vi "get ema report data from imei list file.vi"(8 "error in (no error)":errorcluster) -> (0 "error out":errorcluster, 2 "Rec count":i32, 3 "Array":string[][](array[string]))   [LabVIEW 2013]
uses:
  <vilib>/Utility/file.llb/Read From Spreadsheet File (string).vi
  <vilib>/Utility/file.llb/Write To Spreadsheet File (string).vi
panel:
  in  "Array 2":string[][](array[string])=[["partNumber", "revNumber", "Imei", "Serial", "deviceId", "mfgSerial", "testTimestamp", "simId1", "simId2", "VZWFW", "ATTFW", "moduleBuildVer", "model"]]
  in  "SQL Query":string="SELECT part_number AS partNumber,[PN Rev] AS revNumber,imei AS Imei,deviceserialnumber AS Serial,deviceid0 AS deviceId,btw_sn AS mfgSerial,date_time AS testTimestamp,simid1 AS simId1,simid2 AS simId2,firmware_rev AS VZWFW,deviceid1 AS ATTFW,appfwver AS moduleBuildver,devicename AS model FROM test_data WHERE imei = '"
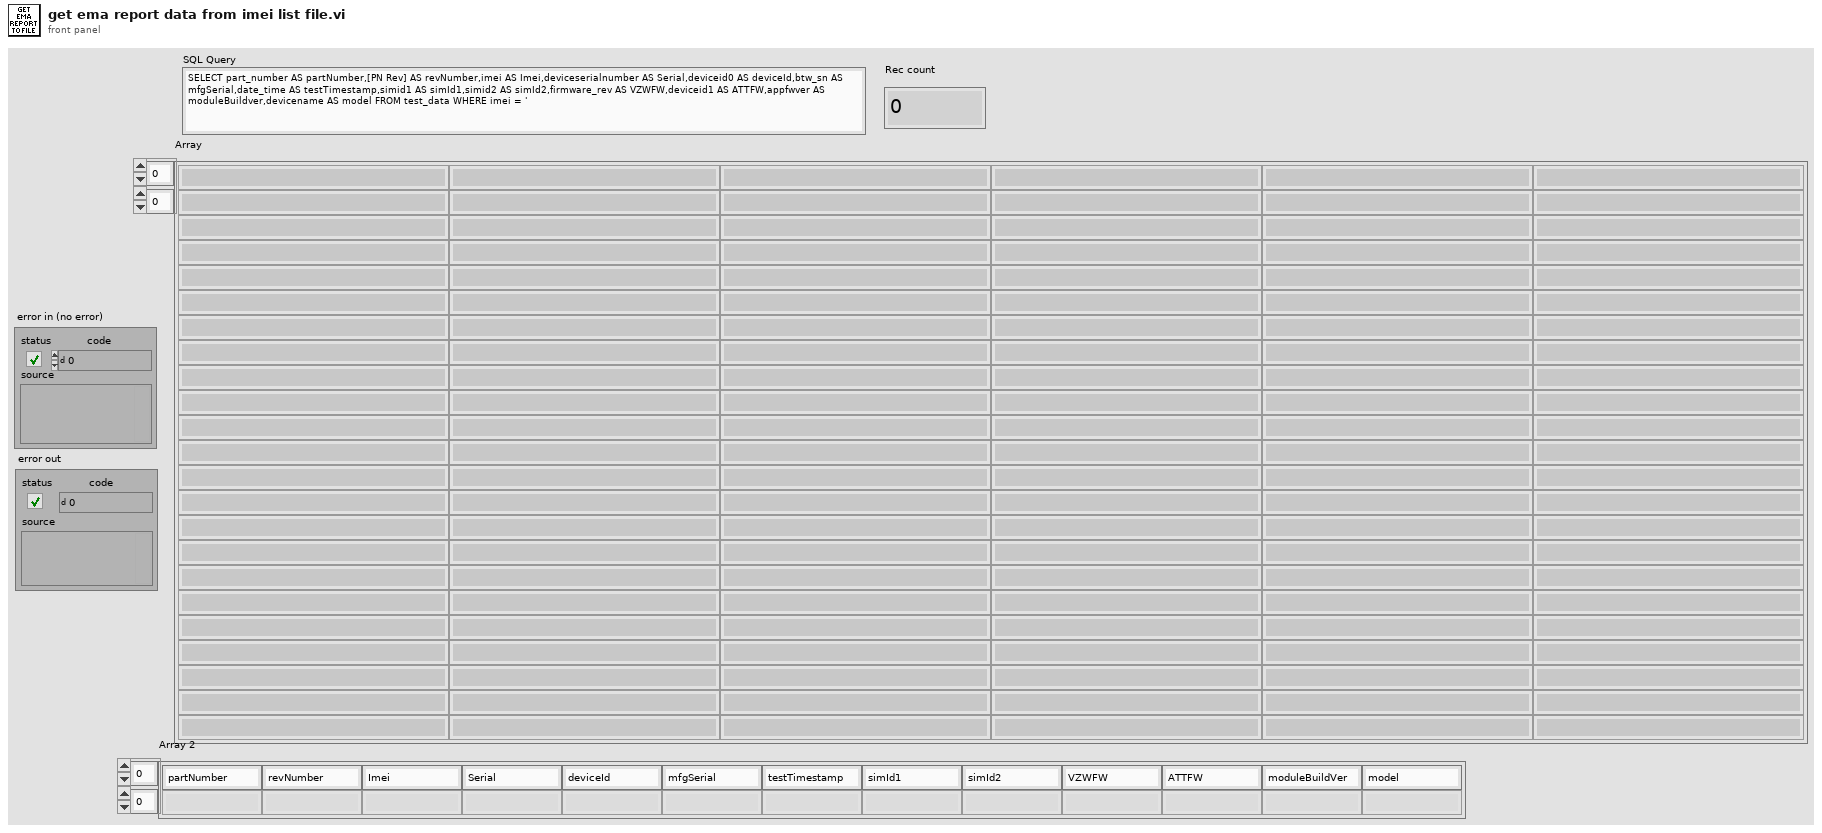
[diagram p1: front panel]
types:
  T1 = enum16{"Query", "Insert", "Select", "Dump Recs", "Get Rec Count", "Get Col Names", "Insert all fields", "Find", "Get last test result", "Get work order qty", "Set work order qty", "Save test report", "Get test report", "Execute query no data", "Select count", "Query and return row 0 col 0"}
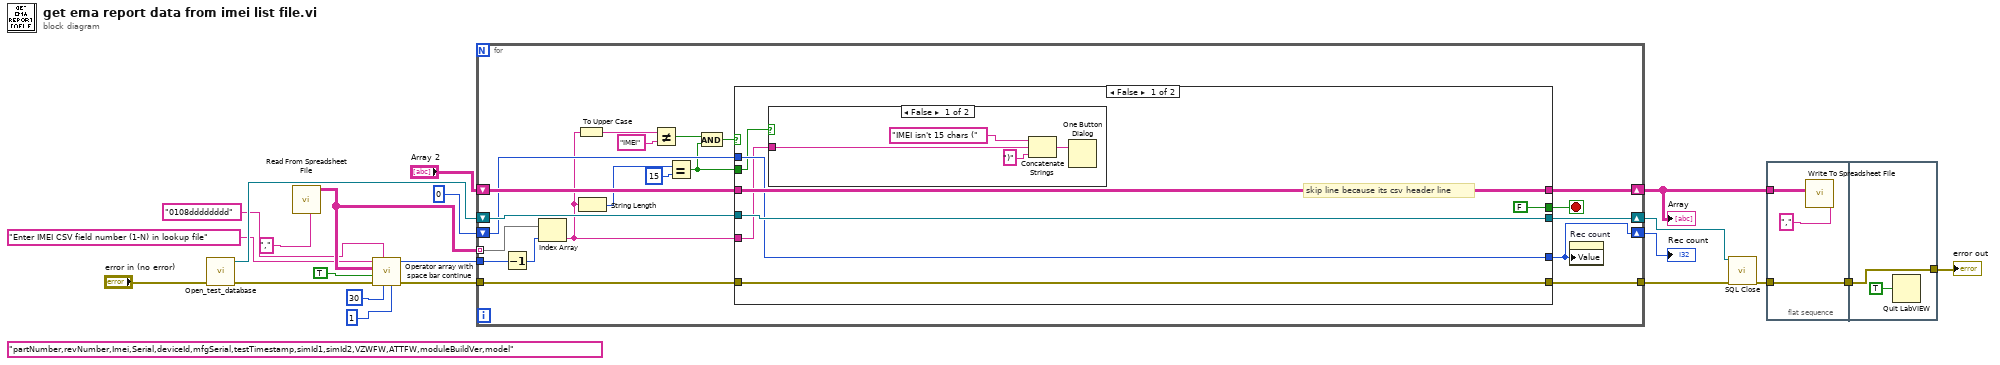
[diagram p0: block diagram]
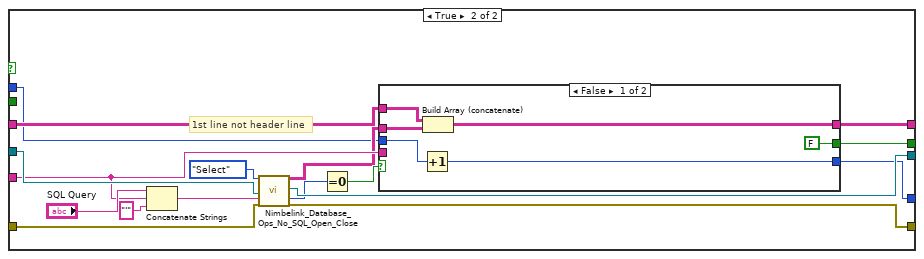
[diagram p3: hidden frame]
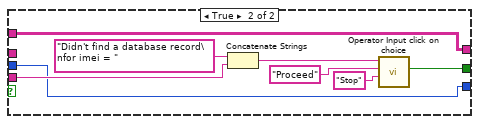
[diagram p4: hidden frame]
diagram:
  (unwired) "partNumber,revNumber,Imei,Serial,deviceId,mfgSerial,testTimestamp,simId1,simId2,VZWFW,ATTFW,moduleBuildVer,model"
  n1 = call "Open_test_database.vi"("error in (no error)"="error in (no error)") -> ("error out"=w6:errorcluster, "SQL conn Refnum out"=w20:refnum<k7>)  [unwired: 9 in]
  n2 = call-poly <vilib>:"Read From Spreadsheet File.vi"("delimiter (\\t)"="," ("delimiter (\\t)")) -> ("all rows"=w13:string[][])  [unwired: 6 in, 4 out]
  n3 = call "Operator array with space bar continue.vi"("Lower limit"=u32 1, "Upper limit"=u32 30, "Data format"="0108dddddddd", "error in (no error)"=w6, "Get decimal response?"=TRUE, "Array"=w13, "Message"="Enter IMEI CSV field number (1-N) in lookup file") -> ("error out"=w5:errorcluster, "Decimal response"=w10:u32)  [unwired: 3 in]
  n4 = for {
    tunnel: w13 -> [w39] mode=indexing
    tunnel: w5 -> [w40]
    shift-right: [w37] -> w1
    shift-left: "Array 2" -> [w38]
    tunnel: [w36] -> w19
    tunnel: w10 -> [w35]
    shift-right: [w28] -> w14
    shift-left: 0 -> [w30]
    shift-right: [w31] -> w15
    shift-left: w20 -> [w41]
    stop <- w29 stop-if-true
    n5 = Decrement(x=w35) -> (x-1=w34:u32)
    n6 = Index Array(array=w39, index=w34) -> (element=w22:string)
    n7 = To Upper Case(1:w22) -> (0:w33:string)
    n8 = String Length(string=w22) -> (length=w27:i32)
    n9 = Not Equal?(x=w33, y="IMEI") -> (x != y?=w25:bool)
    n10 = Equal?(x=w27, y=15) -> (x = y?=w23:bool)
    n11 = And(x=w25, y=w23) -> (x .and. y?=w24:bool)
    n12 = case shown="False" w24 {
      tunnel: w41 -> [w46 w69]
      tunnel: [w46 w68] -> w31
      tunnel: w40 -> [w48 w67]
      tunnel: w22 -> [w42 w61]
      tunnel: w38 -> [w47 w60]
      tunnel: [w47 w59] -> w37
      tunnel: [w48 w57] -> w36
      tunnel: w30 -> [w45 w55]
      tunnel: [w45 w54] -> w28
      tunnel: [FALSE ("button2 clicked?") w53] -> w29
      tunnel: w23 -> [w43 _]
      frame False {
        # "skip line because its csv header line"
        n13 = case shown="False" w43 {
          tunnel: w42 -> [w51 _]
          frame False {
            n14 = Concatenate Strings("IMEI isn't 15 chars (" ("string"), w51, ")" ("string")) -> (w49:string)
            n15 = One Button Dialog(message=w49) -> ()  [unwired: 1 in, 1 out]
          }
          frame True {
          }
        }
      }
      frame True {
        # "1st line not header line"
        n16 = Concatenate Strings("SQL Query", w61, "'" ("string")) -> (w64:string)
        n17 = call "Nimbelink_Database_Ops_No_SQL_Open_Close.vi"("Operation"=T1."Select", "Connection In"=w69, "SQL Query"=w64, "Error in (no error)"=w67) -> ("RecordSet"=w58:string[][], "Connection Out"=w68:refnum<k7>, "Records"=w63:i32, "Error out"=w57:errorcluster)  [unwired: 8 in, 4 out]
        n18 = Equal To 0?(x=w63) -> (x = 0?=w62:bool)
        n19 = case shown="False" w62 {
          tunnel: w61 -> [_ w82]
          tunnel: w60 -> [w75 w81]
          tunnel: [w73 w81] -> w59
          tunnel: w58 -> [w74 _]
          tunnel: w55 -> [w72 w80]
          tunnel: [w71 w80] -> w54
          tunnel: [FALSE ("button2 clicked?") w76] -> w53
          frame False {
            n20 = Increment(x=w72) -> (x+1=w71:i32)
            n21 = Build Array (concatenate)(w75, w74) -> (w73:string[][])
          }
          frame True {
            n22 = Concatenate Strings("Didn't find a database record\nfor imei = " ("message"), w82) -> (w77:string)
            n23 = call "Operator Input click on choice.vi"("button2 text"="Stop", "button1 text"="Proceed", "Operator text"=w77) -> ("button2 clicked?"=w76:bool)  [unwired: 6 in, 2 out]
          }
        }
      }
    }
    n24 = property on="Rec count" class="DigNum (strict)"("Value"=w28) -> ()  [unwired: 2 in, 2 out]
  }
  "Array" <- w1
  "Rec count" <- w14
  n25 = call "SQL Close.vi"("Connection In"=w15, "Error in (no error)"=w19) -> ("Error out"=w3:errorcluster)  [unwired: 17 in]
  n26 = flat-sequence {
    tunnel: w3 -> [w86]
    tunnel: [w86] -> w2
    tunnel: w1 -> [w84]
    tunnel: [w88] -> w4
    tunnel: w2 -> [w88]
    frame #0 {
      n27 = call-poly <vilib>:"Write To Spreadsheet File.vi"("delimiter (\\t)"="," ("delimiter (\\t)"), "2D data"=w84) -> ()  [unwired: 6 in, 1 out]
    }
    frame #1 {
      n28 = Quit LabVIEW(quit? (T)=TRUE) -> ()
    }
  }
  "error out" <- w4
